vi "shape1.vi"() -> ()   [LabVIEW 2020]
panel:
  out "Image Pixels (U8)":u8[][](array[numeric])
  out "Image":T1(plugin-control)
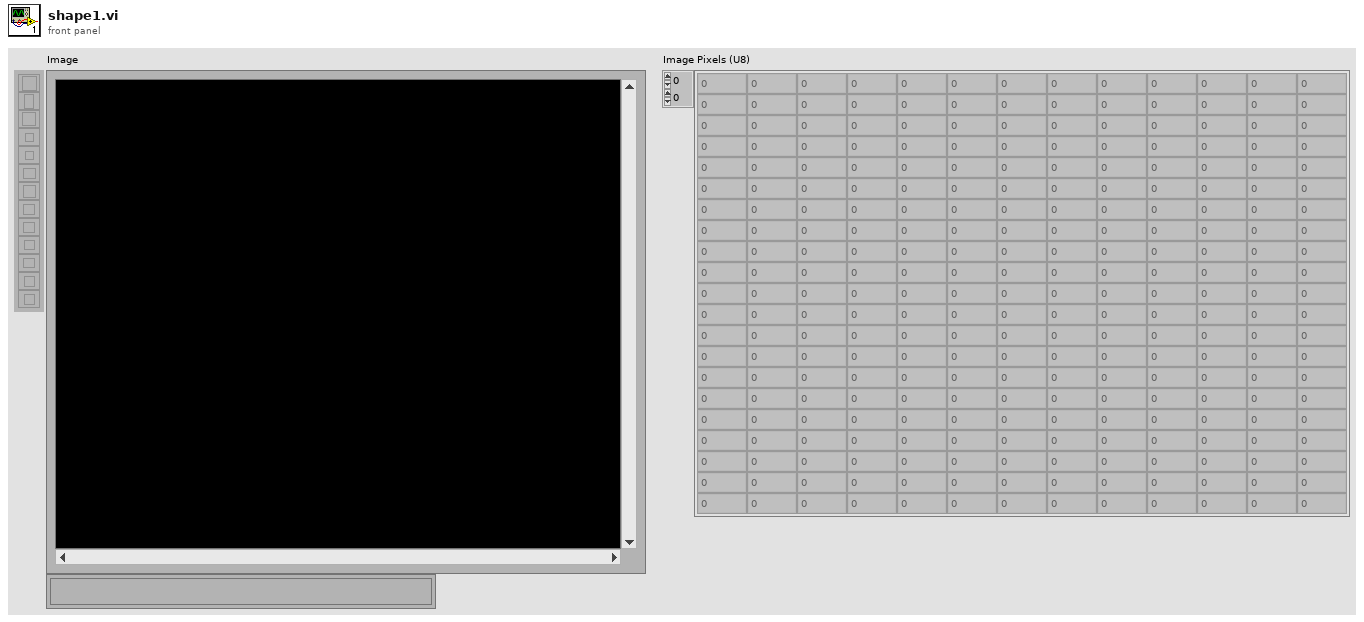
[diagram p1: front panel]
types:
  T1 = typedef "IMAQ Image.ctl" = refnum<image>
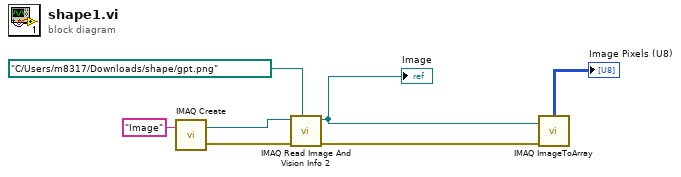
[diagram p0: block diagram]
diagram:
  n1 = call "IMAQ Create"("Image Name"="Image") -> ("New Image"=w5:T1, "error out"=w6:errorcluster)  [unwired: 4 in]
  n2 = call "IMAQ Read Image And Vision Info 2"("File Path"=path "C:/Users/m8317/Downloads/shape/gpt.png", "error in (no error)"=w6, "Image"=w5) -> ("error out"=w3:errorcluster, "Image Out"=w2:T1)  [unwired: 6 in, 1 out]
  "Image" <- w2
  n3 = call "IMAQ ImageToArray"("error in (no error)"=w3, "Image"=w2) -> ("Image Pixels (U8)"=→"Image Pixels (U8)":u8[][])  [unwired: 2 in, 4 out]
